vi "End spectrum measurment.vi"(10 "ContinuousStrobe Out":u32, 11 "Wrapper Out":u32) -> ()   [LabVIEW 2020]
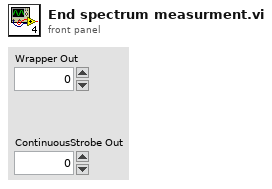
[diagram p1: front panel]
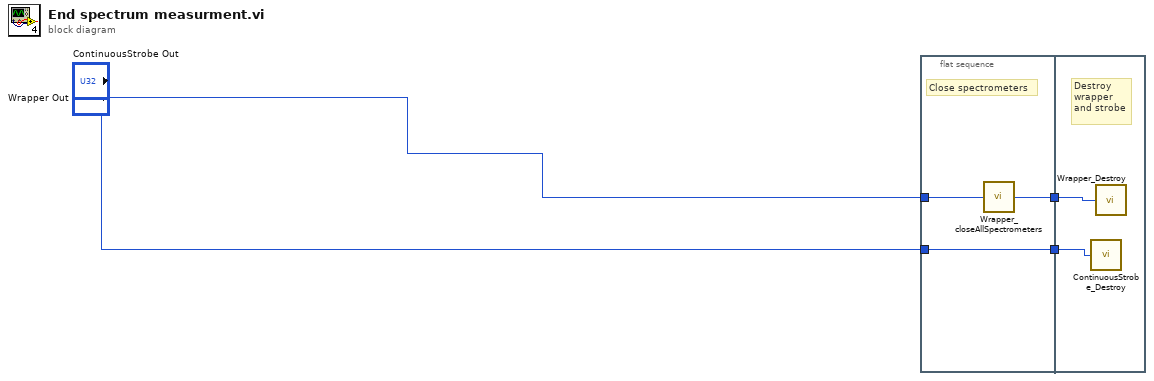
[diagram p0: block diagram]
diagram:
  n1 = flat-sequence {
    tunnel: [w7] -> w4
    tunnel: "Wrapper Out" -> [w6]
    tunnel: [w5] -> w3
    tunnel: "ContinuousStrobe Out" -> [w5]
    tunnel: w4 -> [w9]
    tunnel: w3 -> [w8]
    frame #0 {
      # "Close spectrometers"
      n2 = call "Wrapper_closeAllSpectrometers.vi"("Wrapper In"=w6) -> ("Wrapper Out"=w7:u32)
    }
    frame #1 {
      # "Destroy \nwrapper \nand strobe"
      n3 = call "ContinuousStrobe_Destroy.vi"("ContinuousStrobe"=w8) -> ()
      n4 = call "Wrapper_Destroy.vi"("Wrapper"=w9) -> ()
    }
  }
